vi "Read Defect Identify data.vi"(8 "error in (no error)":errorcluster, 11 "Fiber Auto Collimation state data in":refnum<class "Fiber Auto Collimation state data.lvclass">) -> (0 "error out":errorcluster, 2 "Defect Identify data":cluster{"Image":T1, "Measure Report":string}, 3 "Fiber Auto Collimation state data out":refnum<class "Fiber Auto Collimation state data.lvclass">)   [LabVIEW 2018, in "Fiber Auto Collimation state data.lvclass"]
doc: "This \"LIV test data\" is just a placeholder and example for how real test data might be stored. This accessor plus its data in the state data class private control probably need to be removed or replaced with something to hold test data for the actual station."
uses:
  Fiber Auto Collimation state data.lvclass
  <vilib>/vision/Image Controls.llb/IMAQ Image.ctl
  Fiber Auto Collimation state data.lvclass/Fiber Auto Collimation state data.ctl
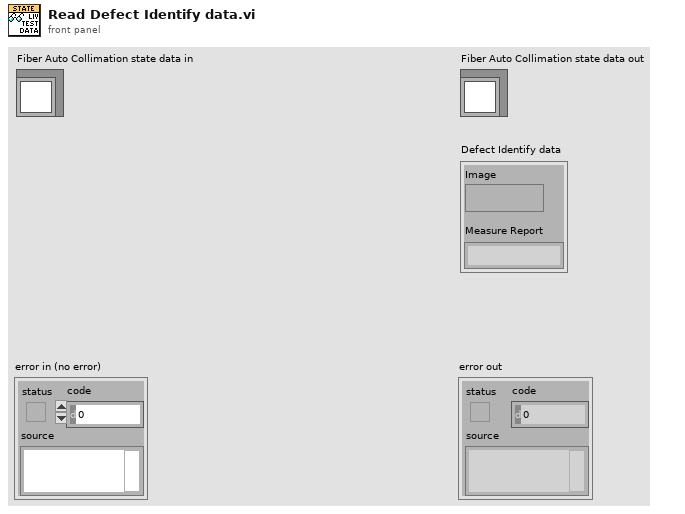
[diagram p1: front panel]
types:
  T1 = typedef "IMAQ Image.ctl" = refnum<image>
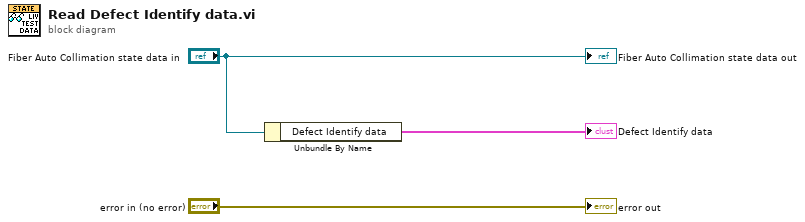
[diagram p0: block diagram]
diagram:
  n1 = Unbundle By Name("Fiber Auto Collimation state data in") -> ("Defect Identify data"=→"Defect Identify data":cluster{"Image":T1, "Measure Report":string})
  "error out" <- "error in (no error)"
  "Fiber Auto Collimation state data out" <- "Fiber Auto Collimation state data in"
